vi "ex_DelDupsFromStringArray.vi"(7 "string array":string[](array[string])) -> (8 "String array without duplicates":string[](array[string]), 10 "List of duplicates (with duplicates)":string[](array[string]))   [LabVIEW 2020]
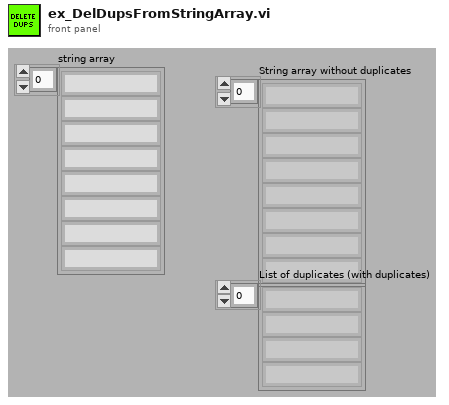
[diagram p1: front panel]
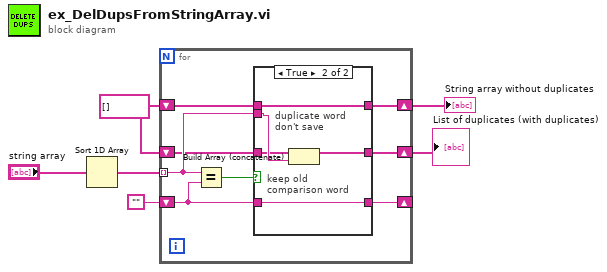
[diagram p0: block diagram]
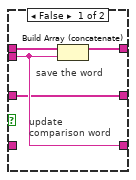
[diagram p2: hidden frame]
diagram:
  w2 = string[] [] ("Array Constant")
  n1 = Sort 1D Array(array="string array") -> (sorted array=w3:string[])
  n2 = for {
    tunnel: w3 -> [w11] mode=indexing
    shift-right: [w10] -> _
    shift-left: "" -> [w9]
    shift-right: [w12] -> w6
    shift-left: w2 -> [w13]
    shift-right: [w8] -> w1
    shift-left: w2 -> [w7]
    n3 = Equal?(x=w11, y=w9) -> (x = y?=w14:bool)
    n4 = case shown="True" w14 {
      tunnel: w13 -> [w18 w20]
      tunnel: [w17 w20] -> w12
      tunnel: w11 -> [w16 w22]
      tunnel: [w16 w23] -> w10
      tunnel: w9 -> [_ w23]
      tunnel: [w15 w21] -> w8
      tunnel: w7 -> [w15 w19]
      frame False {
        # "update\ncomparison word"
        # "save the word"
        n5 = Build Array (concatenate)(w18, w16) -> (w17:string[])
      }
      frame True {
        # "keep old\ncomparison word"
        # "duplicate word\ndon't save"
        n6 = Build Array (concatenate)(w19, w22) -> (w21:string[])
      }
    }
  }
  "String array without duplicates" <- w6
  "List of duplicates (with duplicates)" <- w1
